vi "Read CB air pressure reached.vi"(8 "error in (no error)":errorcluster, 11 "Barometer Bricklet in":refnum<class "Barometer Bricklet.lvclass">) -> (0 "error out":errorcluster, 2 "CB air pressure reached":refnum<user-event>, 3 "Barometer Bricklet out":refnum<class "Barometer Bricklet.lvclass">)   [LabVIEW 2011, in "Tinkerforge.lvlib" / "Barometer Bricklet.lvclass"]
uses:
  Barometer Bricklet.lvclass
  Barometer Bricklet.lvclass/Barometer Bricklet.ctl
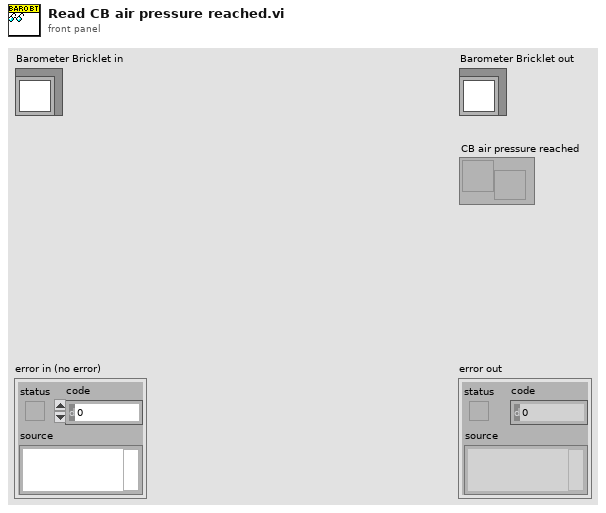
[diagram p1: front panel]
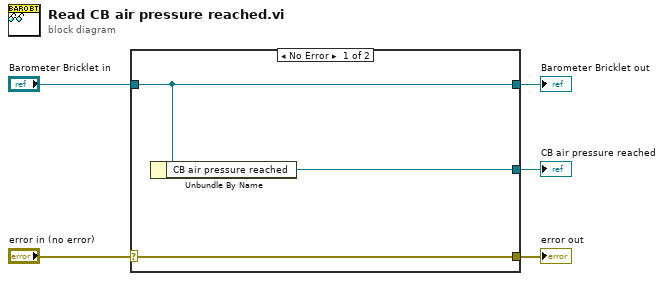
[diagram p0: block diagram]
diagram:
  n1 = case shown="No Error" "error in (no error)" {
    selector: "error in (no error)" -> [w8 w9]
    tunnel: [w8 w9] -> w4
    tunnel: [w7 w10] -> w2
    tunnel: "Barometer Bricklet in" -> [w7 w10]
    tunnel: [w6 _] -> w1
    frame No Error {
      n2 = Unbundle By Name(w7) -> ("CB air pressure reached"=w6:refnum<user-event>)
    }
    frame Error {
    }
  }
  "error out" <- w4
  "Barometer Bricklet out" <- w2
  "CB air pressure reached" <- w1
